vi "Register Event(Single).vi"(8 "error in (no error)":errorcluster, 10 "Event Type":T3=enum."Initialize Finish", 11 "Resister Info":T2) -> (0 "error out":errorcluster)   [LabVIEW 2019, in "FootScan Engine Event.lvlib"]
uses:
  FootScan Engine Event.lvlib
  Event Type.ctl
  <userlib>/JUL/Event Message Module/Event Message Library/Event.ctl
  <userlib>/JUL/Event Message Module/Event Message Library/Event Data Type.ctl
  <userlib>/JUL/Event Message Module/Event Message Library/Event Action.ctl
  <userlib>/JUL/Event Message Module/Event Message Library/Event Message.lvlib
panel:
  # "Input"
  # "Output"
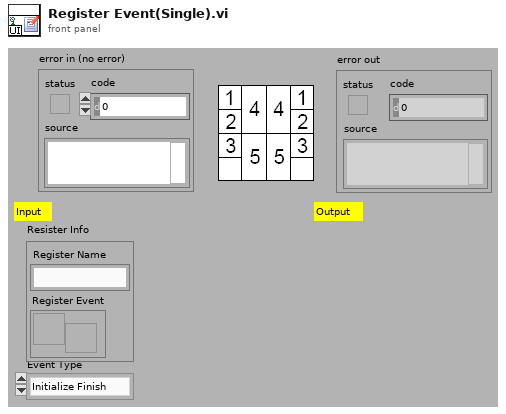
[diagram p1: front panel]
types:
  T1 = typedef "Event Message.lvlib/Event.ctl" = refnum<user-event>
  T2 = cluster{"Register Name":string, "Register Event":T1}
  T3 = typedef "FootScan Engine Event.lvlib/Event Type.ctl" = enum16{"Default", "Initialize Finish", "Button 0 Click", "Exit Click", "Exit"}
  T4 = typedef "Event Action.ctl" = enum16{"Default", "Generate Event", "Register", "Unregister(Customize Event and Register)", "Unregister(All Events In Customize Register)", "Unregister(All Registers In Customize Event)", "Get Register Table"}
  T5 = cluster{"Event Type":T3, "Resister Info":cluster{"Register Name":string, "Register Event":T1}}
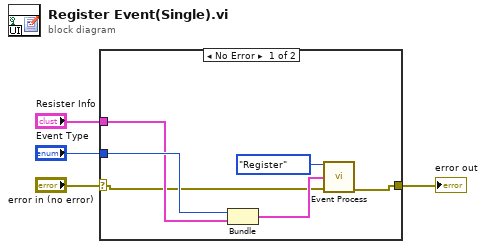
[diagram p0: block diagram]
diagram:
  n1 = case shown="No Error" "error in (no error)" {
    selector: "error in (no error)" -> [w5 w11]
    tunnel: [w9 w11] -> w1
    tunnel: "Event Type" -> [w8 _]
    tunnel: "Resister Info" -> [w7 _]
    frame No Error {
      n2 = Bundle("Event Type"=w8, "Resister Info"=w7) -> (w6:T5)  [unwired: 1 in]
      n3 = call "Event Process.vi"("Event Action"=Event_Action."Register", "Resister Event Data"=w6, "error in (no error)"=w5) -> ("error out"=w9:errorcluster)  [unwired: 11 in, 1 out]
    }
    frame Error {
    }
  }
  "error out" <- w1
